vi "Main.vi"(11 "Module Admin":refnum<class "Delacor_lib_QMH_Module Admin.lvclass">) -> ()   [LabVIEW 2021, in "RT-AutoSequence.lvlib"]
doc: "This template is based off of the Queued Message Handler design pattern and the Queued Message Handler project template that ships with LabVIEW.\n\nThe main difference is that the queue is private to this module and communication between modules is performed via Broadcast and Request events.\n\nRequest events are wrapped in public API methods and are handled in the Event Handling Loop (EHL) of this VI. Any module can register for Broadcast events sent by this module. The EHL generates messages based on user interface actions.\n\nThe Message Handling Loop (MHL) processes messages generated by the EHL, or by other messages. The messages are string values, so new messages can be added easily to the Message Cases case structure in the MHL. Each message cluster can also provide an optional value for Message Data, which is a variant that can be converted to whatever message-specific data is required.\n_____\nBased on DQMH Project Template 7.0.1.1316."
uses:
  RT-AutoSequence.lvlib
  <vilib>/Delacor/Delacor QMH/Libraries/Module Admin_class/Delacor_lib_QMH_Module Admin.lvclass
  Module Data--cluster.ctl
  TCP Engine/Controls/TCP Engine I&O  Interupt Cluster.ctl
  <vilib>/Delacor/Delacor QMH/Libraries/Message Queue_class/Delacor_lib_QMH_Message Queue.lvclass/Delacor_lib_QMH_Message Queue.ctl
  Stop Argument--cluster.ctl
  <vilib>/Delacor/Delacor QMH/Libraries/Module Admin_class/Delacor_lib_QMH_Module Admin.lvclass/Delacor_lib_QMH_Module Admin.ctl
  Configuration Data Argument--cluster.ctl
  Start Auto Sequence Argument--cluster.ctl
  <vilib>/Utility/miscctls.llb/LVPointTypeDef.ctl
  <vilib>/Delacor/Delacor QMH/Libraries/Message Queue_class/Delacor_lib_QMH_Enqueue Message (Single).vi
  <vilib>/Delacor/Delacor QMH/Libraries/Module Admin_class/Delacor_lib_QMH_Get External Launch.vi
  <vilib>/Delacor/Delacor QMH/Libraries/Message Queue_class/Delacor_lib_QMH_Message Queue.lvclass
  TCP Engine/TCP Engine.lvlib
panel:
  out "Numeric":dbl
  out "error out":errorcluster
  out "Status":string
  in  "Simulate MHL Error":bool
  in  "Simulate EHL Error":bool
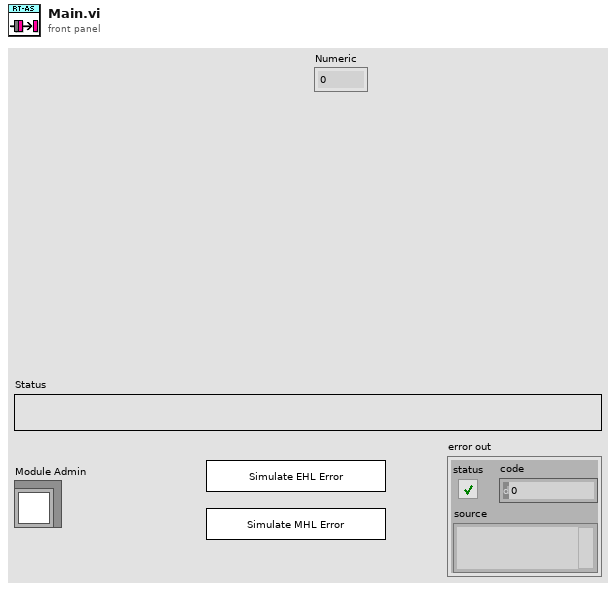
[diagram p1: front panel]
types:
  T1 = typedef "RT-AutoSequence.lvlib/Request Events--cluster.ctl" = cluster{"Stop Module":refnum<user-event>, "Show Panel":refnum<user-event>, "Hide Panel":refnum<user-event>, "Get Module Execution Status":refnum<user-event>, "Show Diagram":refnum<user-event>, "Configuration Data":refnum<user-event>, "Start Auto Sequence":refnum<user-event>}
  T2 = typedef "RT-AutoSequence.lvlib/Module Data--cluster.ctl" = cluster{"Status":string, "DO-Engine Interupt Q":refnum<queue>, "AS-Data's":cluster{"Physical Channel Name":string[], "Identification Name":string[], "Operation":bool[], "Time":dbl[]}, "Start Time":timestamp, "Config Received?":bool, "AS-Time Index":i32}
  T3 = enum32{"invalid lock state", "Not Locked", "Locked (No Password)", "Password-protected"}
  T4 = typedef "RT-AutoSequence.lvlib/Stop Argument--cluster.ctl" = cluster{"Origin":string, "Exit via Stop Module Req?":bool, "Wait for Module to stop?":bool}
  T5 = typedef "RT-AutoSequence.lvlib/Configuration Data Argument--cluster.ctl" = cluster{"AS-Configuration Data":variant}
  T6 = typedef "RT-AutoSequence.lvlib/Start Auto Sequence Argument--cluster.ctl" = cluster{"Start-AS":variant}
  T7 = typedef "LVPointTypeDef.ctl" = cluster{"Horizontal":i16, "Vertical":i16}
  T8 = enum32{"Invalid", "Standard", "Closed", "Hidden", "Minimized", "Maximized"}
  T9 = typedef "TCP Engine.lvlib/TCP Engine I&O  Interupt Cluster.ctl" = cluster{" Stop":bool, "JSON Variant":variant}
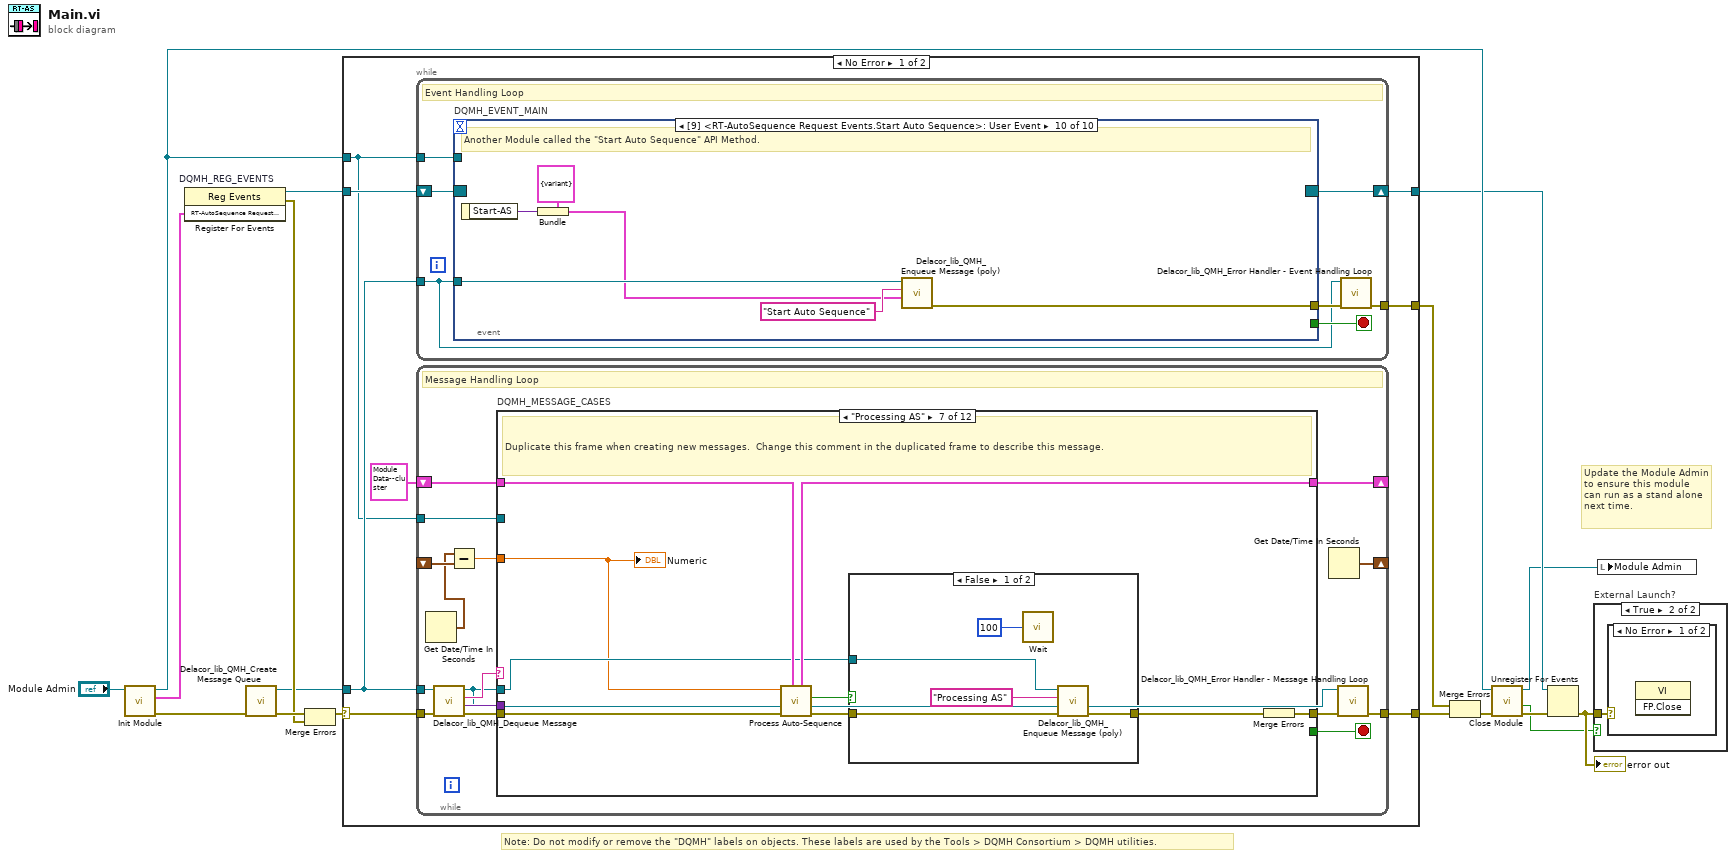
[diagram p0: block diagram]
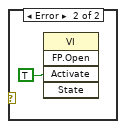
[diagram p3: hidden frame]
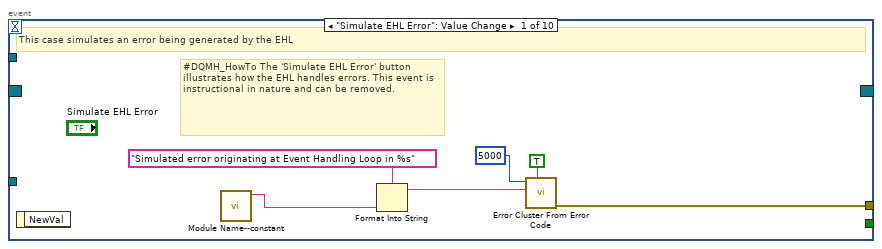
[diagram p4: hidden frame]
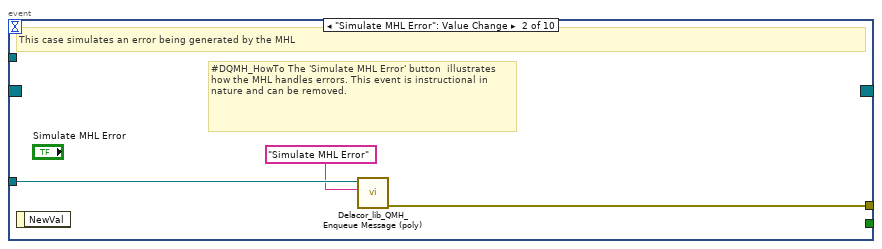
[diagram p5: hidden frame]
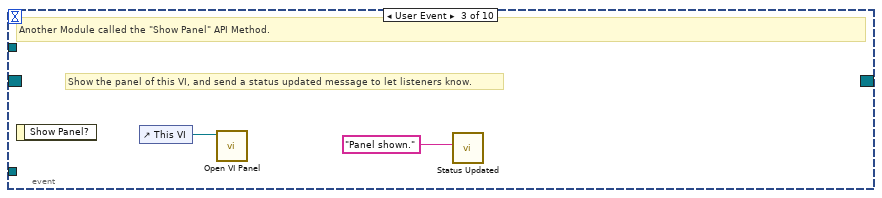
[diagram p6: hidden frame]
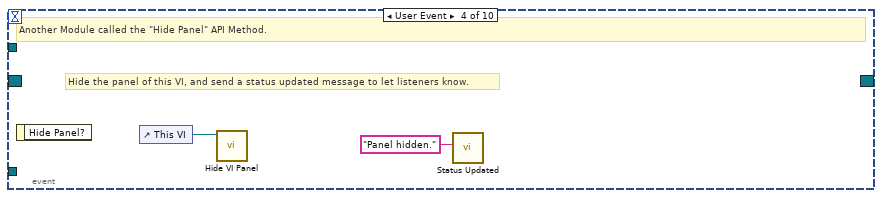
[diagram p7: hidden frame]
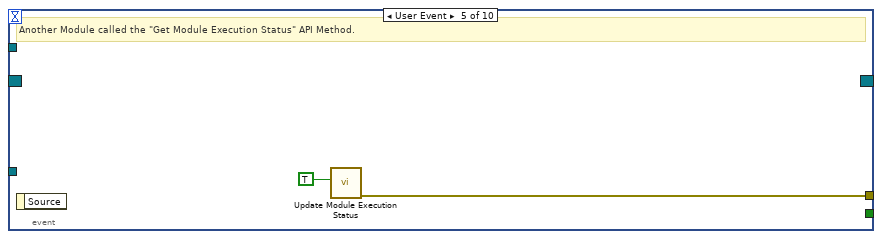
[diagram p8: hidden frame]
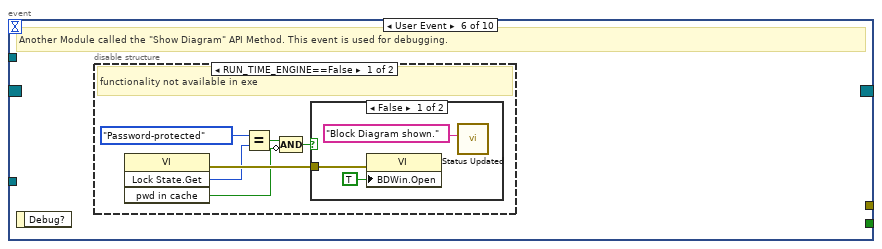
[diagram p9: hidden frame]
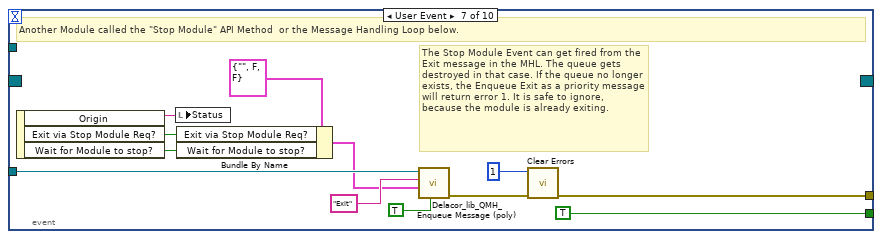
[diagram p12: hidden frame]
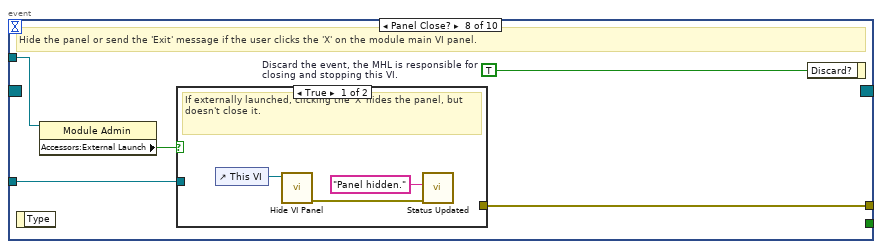
[diagram p13: hidden frame]
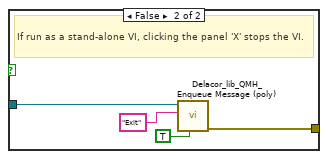
[diagram p14: hidden frame]
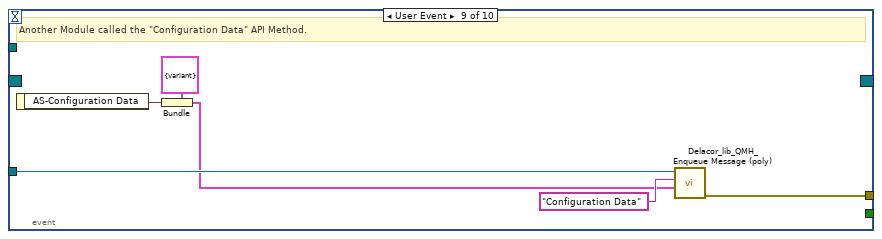
[diagram p15: hidden frame]
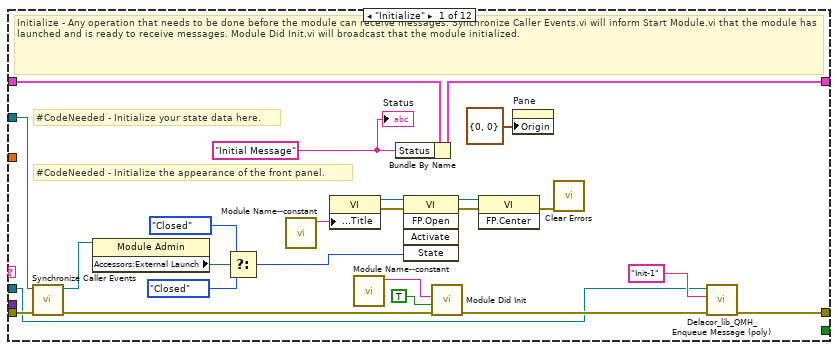
[diagram p16: hidden frame]
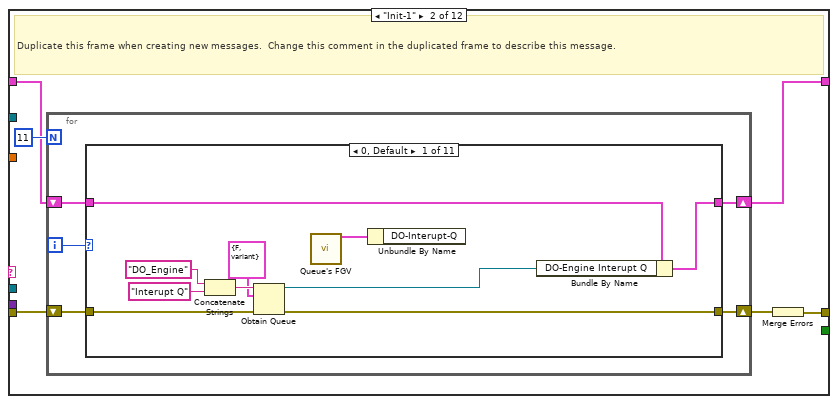
[diagram p17: hidden frame]
diagram:
  # "Note: Do not modify or remove the \"DQMH\" labels on objects. These labels are used by the Tools > DQMH Consortium > DQMH utilities."
  # "Update the Module Admin to ensure this module can run as a stand alone next time."
  n1 = call "Init Module.vi"("Singleton Module Admin in"="Module Admin") -> ("error out"=w16:errorcluster, "RT-AutoSequence Request Events"=w5:T1, "Singleton Module Admin out"=w8:refnum<class "Delacor_lib_QMH_Module Admin.lvclass">)  [unwired: 8 in]
  n2 = register-events "DQMH_REG_EVENTS"(w5) -> (reference out=w6:refnum<event-registration>, error out=w9:errorcluster)  [unwired: 2 in]
  n3 = call <vilib>:"Delacor_lib_QMH_Create Message Queue.vi"("error in"=w16) -> ("error out"=w11:errorcluster, "Message Queue"=w4:refnum<class "Delacor_lib_QMH_Message Queue.lvclass">)  [unwired: 9 in]
  n4 = Merge Errors(w11, w9) -> (w10:errorcluster)
  n5 = case shown="No Error" w10 {
    selector: w10 -> [w23 w276]
    tunnel: [w25 w275] -> w17
    tunnel: [w22 w274] -> w7
    tunnel: w6 -> [w21 w274]
    tunnel: w4 -> [w20 w269]
    tunnel: [w24 _] -> w14
    tunnel: w8 -> [w19 w270]
    frame No Error {
      n6 = while {
        tunnel: w20 -> [w26]
        shift-right: [w29] -> w22
        shift-left: w21 -> [w30]
        tunnel: [w31] -> w24
        tunnel: w19 -> [w27]
        stop <- w28 stop-if-true
        # "Event Handling Loop"
        n7 = event "DQMH_EVENT_MAIN" shown="[9] <RT-AutoSequence Request Events.Start Auto Sequence>: User Event" {
          selector: w30 -> [_ _ _ _ _ _ _ _ _ _]
          dyn-events: [_ _ _ _ _ _ _ _ _ _] -> w29
          timeout: _ -> [_ _ _ _ _ _ _ _ _ _]
          tunnel: [_ _ _ _ _ _ TRUE ("Discard?") _ _ _] -> w28
          tunnel: w26 -> [_ w40 _ _ _ _ w64 w71 w86 w92]
          tunnel: [w38 w41 _ _ w47 _ w67 w73 w81 w87] -> w32
          tunnel: w27 -> [_ _ _ _ _ _ _ w70 _ _]
          event "Simulate EHL Error": Value Change {
            # "#DQMH_HowTo The 'Simulate EHL Error' button  illustrates how the EHL handles errors. This event is instructional in nature and can be removed."
            # "This case simulates an error being generated by the EHL"
            n8 = event-data() -> ()  [unwired: 1 in, 1 out]
            n9 = call "Module Name--constant.vi"() -> ("Module Name"=w35:string)  [unwired: 11 in]
            n10 = Format Into String(format string="Simulated error originating at Event Handling Loop in %s", w35) -> (resulting string=w36:string)  [unwired: 2 in, 1 out]
            n11 = call <vilib>:"Error Cluster From Error Code.vi"("show call chain? (False)"=TRUE, "error message (\"\")"=w36, "error code (0)"=5000) -> ("error out"=w38:errorcluster)  [unwired: 6 in]
          }
          event "Simulate MHL Error": Value Change {
            # "#DQMH_HowTo The 'Simulate MHL Error' button  illustrates how the MHL handles errors. This event is instructional in nature and can be removed."
            # "This case simulates an error being generated by the MHL"
            n12 = event-data() -> ()  [unwired: 1 in, 1 out]
            n13 = call-poly <vilib>:"Delacor_lib_QMH_Enqueue Message (poly).vi"("Message"="Simulate MHL Error", "Message Queue in"=w40) -> ("error out"=w41:errorcluster)  [unwired: 8 in, 1 out]
          }
          event User Event {
            # "Show the panel of this VI, and send a status updated message to let listeners know."
            # "Another Module called the \"Show Panel\" API Method."
            n14 = event-data() -> ()  [unwired: 1 in, 1 out]
            n15 = control-ref of="This VI"() -> (w43:refnum<vi>)
            n16 = call "Open VI Panel.vi"("VI"=w43) -> ()  [unwired: 10 in, 1 out]
            n17 = call "Status Updated.vi"("Status"="Panel shown." ("format string")) -> ()  [unwired: 10 in, 1 out]
          }
          event User Event {
            # "Hide the panel of this VI, and send a status updated message to let listeners know."
            # "Another Module called the \"Hide Panel\" API Method."
            n18 = event-data() -> ()  [unwired: 1 in, 1 out]
            n19 = control-ref of="This VI"() -> (w45:refnum<vi>)
            n20 = call "Hide VI Panel.vi"("VI"=w45) -> ()  [unwired: 10 in, 1 out]
            n21 = call "Status Updated.vi"("Status"="Panel hidden." ("format string")) -> ()  [unwired: 10 in, 1 out]
          }
          event User Event {
            # "Another Module called the \"Get Module Execution Status\" API Method."
            n22 = event-data() -> ()  [unwired: 1 in, 1 out]
            n23 = call "Update Module Execution Status.vi"("Running?"=TRUE) -> ("error out"=w47:errorcluster)  [unwired: 10 in]
          }
          event User Event {
            # "Another Module called the \"Show Diagram\" API Method. This event is used for debugging."
            n24 = event-data() -> ()  [unwired: 1 in, 1 out]
            n25 = disable-structure shown="RUN_TIME_ENGINE==False" {
              frame condition #0 (active) {
                # "functionality not available in exe"
                n26 = invoke on="Invoke Node" class="VI" method="Lock State.Get"() -> (error out=w53:errorcluster, "Get Lock State"=w52:T3, "pwd in cache"=w49:bool)  [unwired: 4 in, 1 out]
                n27 = Equal?(x=T3."Password-protected", y=w52) -> (x = y?=w50:bool)
                n28 = Compound Arithmetic op=AND(w50, invert w49) -> (w48:bool)
                n29 = case shown="False" w48 {
                  tunnel: w53 -> [w56 _]
                  frame False {
                    n30 = property on="Property Node" class="VI"(error in=w56, "BDWin.Open"=TRUE ("Block Diagram Window:Open")) -> ()  [unwired: 1 in, 2 out]
                    n31 = call "Status Updated.vi"("Status"="Block Diagram shown." ("format string")) -> ()  [unwired: 10 in, 1 out]
                  }
                  frame True {
                    # "Password-protected VI, and the password is not in the cache. Do not show the diagram."
                  }
                }
              }
              frame condition #1 {
              }
            }
          }
          event User Event {
            # "The Stop Module Event can get fired from the Exit message in the MHL. The queue gets destroyed in that case. If the queue no longer exists, the Enqueue Exit as a priority message will return error 1. It is safe to ignore, because the module is already exiting."
            # "Another Module called the \"Stop Module\" API Method  or the Message Handling Loop below."
            n32 = event-data() -> ("Origin"=w63:string, "Exit via Stop Module Req?"=w59:bool, "Wait for Module to stop?"=w58:bool)  [unwired: 1 in]
            n33 = local write "Status"(w63) -> ()
            n34 = Bundle By Name(cluster=T4 {"Origin"="", "Exit via Stop Module Req?"=FALSE, "Wait for Module to stop?"=FALSE} ("Stop Argument"), "Exit via Stop Module Req?"=w59, "Wait for Module to stop?"=w58) -> (w57:T4)
            n35 = call-poly <vilib>:"Delacor_lib_QMH_Enqueue Message (poly).vi"("Priority Message? (F)"=TRUE, "Message Data"=w57, "Message"="Exit", "Message Queue in"=w64) -> ("error out"=w68:errorcluster)  [unwired: 6 in, 1 out]
            n36 = call <vilib>:"Clear Errors.vi"("error in (no error)"=w68, "specific error code to clear (0: all)"=1) -> ("error out"=w67:errorcluster)  [unwired: 4 in, 1 out]
          }
          event Panel Close? {
            w72 = TRUE  # Discard the event, the MHL is responsible for closing and stopping this VI.
            # "Hide the panel or send the 'Exit' message if the user clicks the 'X' on the module main VI panel."
            n37 = event-data() -> ()  [unwired: 1 in, 1 out]
            n38 = property on="Property Node" class="Module Admin"(reference=w70) -> ("Accessors:External Launch"=w69:bool)  [unwired: 1 in, 2 out]
            n39 = case shown="True" w69 {
              tunnel: w71 -> [_ w79]
              tunnel: [_ w80] -> w73
              frame True {
                # "If externally launched, clicking the 'X' hides the panel, but doesn't close it."
                n40 = control-ref of="This VI"() -> (w76:refnum<vi>)
                n41 = call "Hide VI Panel.vi"("VI"=w76) -> ("error out"=w74:errorcluster)  [unwired: 10 in]
                n42 = call "Status Updated.vi"("error in"=w74, "Status"="Panel hidden." ("format string")) -> ()  [unwired: 9 in, 1 out]
              }
              frame False {
                # "If run as a stand-alone VI, clicking the panel 'X' stops the VI."
                n43 = call-poly <vilib>:"Delacor_lib_QMH_Enqueue Message (poly).vi"("Priority Message? (F)"=TRUE, "Message"="Exit", "Message Queue in"=w79) -> ("error out"=w80:errorcluster)  [unwired: 7 in, 1 out]
              }
            }
            n44 = event-data ("Event Filter Node")("Discard?"=w72) -> ()  [unwired: 1 in, 1 out]
          }
          event User Event {
            # "Another Module called the \"Configuration Data\" API Method."
            n45 = event-data() -> ("AS-Configuration Data"=w82:variant)  [unwired: 1 in]
            n46 = Bundle(cluster=T5 {"AS-Configuration Data"=variant} ("Configuration Data Argument"), "AS-Configuration Data"=w82) -> (w83:T5)
            n47 = call-poly <vilib>:"Delacor_lib_QMH_Enqueue Message (poly).vi"("Message Data"=w83, "Message"="Configuration Data", "Message Queue in"=w86) -> ("error out"=w81:errorcluster)  [unwired: 7 in, 1 out]
          }
          event User Event {
            # "Another Module called the \"Start Auto Sequence\" API Method."
            n48 = event-data() -> ("Start-AS"=w88:variant)  [unwired: 1 in]
            n49 = Bundle(cluster=T6 {"Start-AS"=variant} ("Start Auto Sequence Argument"), "Start-AS"=w88) -> (w89:T6)
            n50 = call-poly <vilib>:"Delacor_lib_QMH_Enqueue Message (poly).vi"("Message Data"=w89, "Message"="Start Auto Sequence", "Message Queue in"=w92) -> ("error out"=w87:errorcluster)  [unwired: 7 in, 1 out]
          }
        }
        n51 = call-dynamic "Delacor_lib_QMH_Error Handler - Event Handling Loop.vi"("error in"=w32, "Message Queue in"=w26) -> ("dup error in"=w31:errorcluster)  [unwired: 8 in, 1 out]
      }
      n52 = while {
        tunnel: w20 -> [w97]
        shift-right: [w105] -> _
        shift-left: T2 {"Status"="", "DO-Engine Interupt Q"=refnum, "AS-Data's"={"Physical Channel Name"=[], "Identification Name"=[], "Operation"=[], "Time"=[]}, "Start Time"=timestamp(0 s since 1904-01-01), "Config Received?"=FALSE, "AS-Time Index"=0} ("Data Cluster") -> [w106]
        tunnel: w23 -> [w108]
        tunnel: [w100] -> w25
        tunnel: w19 -> [w101]
        shift-right: [w94] -> _
        shift-left: _ -> [w96]
        stop <- w104 stop-if-true
        # "Message Handling Loop"
        n53 = Get Date/Time In Seconds() -> (seconds since 1Jan1904=w93:timestamp)
        n54 = call-dynamic "Delacor_lib_QMH_Dequeue Message.vi"("error in"=w108, "Message Queue in"=w97) -> ("error out"=w107:errorcluster, "Message Data"=w102:variant, "Message"=w103:string, "Message Queue out"=w98:refnum<class "Delacor_lib_QMH_Message Queue.lvclass">)  [unwired: 6 in]
        n55 = Subtract(x=w93, y=w96) -> (x-y=w95:dbl)
        n56 = case "DQMH_MESSAGE_CASES" shown="\"Processing AS\"" w103 {
          selector: w103 -> [_ _ _ _ _ _ _ _ _ _ _ w264]
          tunnel: w98 -> [w109 _ _ _ w189 _ w203 _ _ w230 w252 _]
          tunnel: w107 -> [w130 w134 w175 w186 w197 w200 w207 w217 w226 w237 w258 w267]
          tunnel: [w110 w138 w175 w179 w187 w199 w209 w217 w225 w233 w253 w268] -> w99
          tunnel: w106 -> [w120 w136 w174 w178 w193 w198 w208 w216 w223 w232 w251 w265]
          tunnel: [w119 w133 w174 w182 w192 w198 w206 w216 w223 w232 w251 w265] -> w105
          tunnel: [_ _ _ _ _ _ _ _ _ _ w250 _] -> w104
          tunnel: w102 -> [_ _ _ w185 w196 _ _ _ _ w231 w249 _]
          tunnel: w101 -> [w121 _ _ _ _ _ _ _ _ w229 w244 _]
          tunnel: w95 -> [_ _ _ _ _ _ w201 _ _ _ _ _]
          frame "Initialize" {
            w115 = "Initial Message" ("Initial Message")
            # "#CodeNeeded - Initialize the appearance of the front panel."
            # "#CodeNeeded - Initialize your state data here."
            # "Initialize - Any operation that needs to be done before the module can receive messages. Synchronize Caller Events.vi will inform Start Module.vi that the module has launched and is ready to receive messages. Module Did Init.vi will broadcast that the module initialized."
            n57 = call "Synchronize Caller Events.vi"("error in"=w130, "Singleton Module Admin in"=w121) -> ("error out"=w129:errorcluster, "Singleton Module Admin out"=w116:refnum<class "Delacor_lib_QMH_Module Admin.lvclass">)  [unwired: 8 in]
            n58 = property on="Property Node" class="Module Admin"(reference=w116) -> ("Accessors:External Launch"=w125:bool)  [unwired: 1 in, 2 out]
            n59 = Select(t=T8."Closed" ("State"), s=w125, f=T8."Closed" ("State")) -> (s? t:f=w122:T8)
            n60 = call "Module Name--constant.vi"() -> ("Module Name"=w128:string)  [unwired: 11 in]
            n61 = property on="Property Node" class="VI"("Front Panel.Title"=w128) -> (reference out=w127:refnum<vi>, error out=w132:errorcluster)  [unwired: 2 in]
            n62 = call "Module Name--constant.vi"() -> ("Module Name"=w117:string)  [unwired: 11 in]
            n63 = Bundle By Name(cluster=w120, "Status"=w115) -> (w119:T2)
            n64 = invoke on="Invoke Node" class="VI" method="FP.Open"(reference=w127, error in=w132, "State"=w122) -> (reference out=w126:refnum<vi>, error out=w131:errorcluster)  [unwired: 2 in, 3 out]
            n65 = call "Module Did Init.vi"("error in"=w129, "Initialized?"=TRUE, "Origin"=w117) -> ("error out"=w111:errorcluster)  [unwired: 8 in]
            n66 = invoke on="Invoke Node" class="VI" method="FP.Center"(reference=w126, error in=w131) -> (error out=w113:errorcluster)  [unwired: 1 in, 2 out]
            n67 = property on="Pane" class="Pane"("Origin"=T7 {"Horizontal"=0, "Vertical"=0}) -> ()  [unwired: 2 in, 2 out]
            n68 = call <vilib>:"Clear Errors.vi"("error in (no error)"=w113) -> ()  [unwired: 5 in, 2 out]
            n69 = call-poly <vilib>:"Delacor_lib_QMH_Enqueue Message (poly).vi"("error in"=w111, "Message"="Init-1", "Message Queue in"=w109) -> ("error out"=w110:errorcluster)  [unwired: 7 in, 1 out]
            "Status" <- w115
          }
          frame "Init-1" {
            # "Duplicate this frame when creating new messages.  Change this comment in the duplicated frame to describe this message."
            n70 = for {
              N: 11 -> [_]
              shift-right: [w142] -> w133
              shift-left: w136 -> [w143]
              shift-right: [w140] -> w135
              shift-left: w134 -> [w139]
              i -> [w141]
              n71 = case shown="0, Default" w141 {
                tunnel: w143 -> [w147 w155 w157 w159 w161 w163 w165 w167 w169 w171 w173]
                tunnel: [w146 w155 w157 w159 w161 w163 w165 w167 w169 w171 w173] -> w142
                tunnel: [w148 w154 w156 w158 w160 w162 w164 w166 w168 w170 w172] -> w140
                tunnel: w139 -> [w149 w154 w156 w158 w160 w162 w164 w166 w168 w170 w172]
                frame 0, Default {
                  n72 = Concatenate Strings("DO_Engine" ("Engine Name"), "Interupt Q" ("string")) -> (w153:string)
                  n73 = Obtain Queue(name (unnamed)=w153, element data type=T9 {" Stop"=FALSE, "JSON Variant"=variant(string "")} ("I/O  Interupt Cluster"), error in (no error)=w149) -> (queue out=w144:refnum<queue>, error out=w148:errorcluster)  [unwired: 2 in, 1 out]
                  n74 = call "Queue's FGV.vi"() -> ("Cluster"=w145:cluster{"DO-Interupt-Q":refnum<queue>})  [unwired: 14 in, 1 out]
                  n75 = Unbundle By Name(w145) -> ()  [unwired: 1 out]
                  n76 = Bundle By Name(cluster=w147, "DO-Engine Interupt Q"=w144) -> (w146:T2)
                }
                frame 1 {
                }
                frame 2 {
                }
                frame 3 {
                }
                frame 4 {
                }
                frame 5 {
                }
                frame 6 {
                }
                frame 7 {
                }
                frame 8 {
                }
                frame 9 {
                }
                frame 10 {
                }
              }
            }
            n77 = Merge Errors(w135) -> (w138:errorcluster)
          }
          frame "---Module Specific---" {
            # "Separator -- The following cases handle messages specific to this Module."
          }
          frame "Configuration Data" {
            # "This Request event will send the AutoSequence configuration which has been received from the Host through TCP-IP module to AutoSequence Module."
            n78 = Variant To Data(error in=w186, type=T5 {"AS-Configuration Data"=variant} ("Configuration Data Argument"), Variant=w185) -> (data=w183:T5, error out=w180:errorcluster)
            n79 = Unbundle By Name(w183) -> ("AS-Configuration Data"=w181:variant)
            n80 = Bundle By Name(cluster=w178, "Config Received?"=TRUE) -> (w177:T2)
            n81 = call "Configure Timing's.vi"("Data Cluster In"=w177, "error in (no error)"=w180, "Configuration Data"=w181) -> ("error out"=w179:errorcluster, "Data Cluster Out"=w182:T2)  [unwired: 7 in]
          }
          frame "Start Auto Sequence" {
            # "This Request Event will give the start command which has been received from the Host using TCP-IP module to the Auto Sequence Module."
            n82 = Variant To Data(error in=w197, type=T6 {"Start-AS"=variant} ("Start Auto Sequence Argument"), Variant=w196) -> (data=w194:T6, error out=w188:errorcluster)
            n83 = Unbundle By Name(w194) -> ()  [unwired: 1 out]
            n84 = call-poly <vilib>:"Delacor_lib_QMH_Enqueue Message (poly).vi"("error in"=w188, "Message"="Processing AS", "Message Queue in"=w189) -> ("error out"=w187:errorcluster)  [unwired: 7 in, 1 out]
            n85 = Get Date/Time In Seconds() -> (seconds since 1Jan1904=w191:timestamp)
            n86 = Bundle By Name(cluster=w193, "Start Time"=w191) -> (w192:T2)
          }
          frame "---Copy This Frame---" {
            # "Duplicate this frame when creating new messages.  Change this comment in the duplicated frame to describe this message."
            n87 = Merge Errors(w200) -> (w199:errorcluster)
          }
          frame "Processing AS" {
            # "Duplicate this frame when creating new messages.  Change this comment in the duplicated frame to describe this message."
            n88 = call "Process Auto-Sequence.vi"("Data Cluster In"=w208, "error in"=w207, "y"=w201) -> ("error out"=w204:errorcluster, "Again Process?"=w205:bool, "Data Cluster Out"=w206:T2)  [unwired: 6 in]
            n89 = case shown="False" w205 {
              tunnel: w204 -> [w213 w215]
              tunnel: w203 -> [w214 _]
              tunnel: [w212 w215] -> w202
              frame False {
                n90 = call "Wait"("Count(mSec)"=u32 100 ("milliseconds to wait")) -> ()  [unwired: 1 out]
                n91 = call-poly <vilib>:"Delacor_lib_QMH_Enqueue Message (poly).vi"("error in"=w213, "Message"="Processing AS", "Message Queue in"=w214) -> ("error out"=w212:errorcluster)  [unwired: 7 in, 1 out]
              }
              frame True {
              }
            }
            n92 = Merge Errors(w202) -> (w209:errorcluster)
            "Numeric" <- w201
          }
          frame "---Exit and Error Handling---" {
            # "Separator - The following cases handle errors and exit messages."
          }
          frame "Simulate MHL Error" {
            # "#DQMH_HowTo The 'Simulate MHL Error' button  illustrates how the MHL handles errors. This event is instructional in nature and can be removed."
            # "Simulate an error occurring at the MHL"
            n93 = call "Module Name--constant.vi"() -> ("Module Name"=w219:string)  [unwired: 11 in]
            n94 = Format Into String(format string="Simulated error originating at Message Handling Loop in %s", w219) -> (resulting string=w220:string)  [unwired: 2 in, 1 out]
            n95 = call <vilib>:"Error Cluster From Error Code.vi"("show call chain? (False)"=TRUE, "error message (\"\")"=w220, "error code (0)"=5001) -> ("error out"=w224:errorcluster)  [unwired: 6 in]
            n96 = Merge Errors(w226, w224) -> (w225:errorcluster)
          }
          frame "Error" {
            # "#CodeRecommended - If the module is running in standalone mode (External Launch = FALSE), this code will pop up an error dialog and call the 'Exit' message if an error occurs. Add more fine-grained error management here."
            # "Error - Check the error message data and respond accordingly. This message is sent by the \"Error Handler\" VIs at the end of each loop in this application."
            n97 = property on="Property Node" class="Module Admin"(reference=w229) -> ("Accessors:External Launch"=w228:bool)  [unwired: 1 in, 2 out]
            n98 = Variant To Data(error in=w237, type=errorcluster {"status"=FALSE, "code"=0, "source"=""} ("error constant"), Variant=w231) -> (data=w227:errorcluster, error out=w235:errorcluster)
            n99 = local write "error out"(w227) -> ()
            n100 = call "Error Reported.vi"("Error"=w227) -> ()  [unwired: 10 in, 1 out]
            n101 = case shown="False" w228 {
              tunnel: [w242 _] -> w234
              tunnel: w230 -> [w240 _]
              tunnel: w227 -> [w241 _]
              frame False {
                n102 = disable-structure shown="Default" {
                  disable-tunnel: w241 -> [w243 _]
                  frame condition #0 (active) {
                    # "If the module is running standalone, then pop up an error dialog and call the \"Exit\" message."
                    n103 = call <vilib>:"Simple Error Handler.vi"("error in (no error)"=w243) -> ()  [unwired: 4 in, 5 out]
                  }
                  frame condition #1 {
                    # "To prevent the Simple Error Handler VI from being loaded (e.g. when deploying to a Real-Time target), add the Conditional Disable Symbol \"DQMH_Disable_SEH\" to your project and set it to TRUE."
                  }
                }
                n104 = call-poly <vilib>:"Delacor_lib_QMH_Enqueue Message (poly).vi"("Priority Message? (F)"=TRUE, "Message"="Exit", "Message Queue in"=w240) -> ("error out"=w242:errorcluster)  [unwired: 7 in, 1 out]
              }
              frame True {
                # "If the module was launched externally, calling the Error Reported broadcast VI is the only action performed by the \"Error\" message. The module's caller can then process the error appropriately."
              }
            }
            n105 = Merge Errors(w235, w234) -> (w233:errorcluster)
          }
          frame "Exit" {
            w248 = 91  # 91: not all Exit messages will have an argument
            w250 = TRUE  # Stop the VI
            # "Release the message queue reference"
            # "#CodeNeeded - Add any required cleanup code here."
            # "Exit - Exit the application."
            n106 = Variant To Data(error in=w258, type=T4 {"Origin"="", "Exit via Stop Module Req?"=FALSE, "Wait for Module to stop?"=FALSE} ("Stop Argument"), Variant=w249) -> (data=w246:T4, error out=w255:errorcluster)
            n107 = call <vilib>:"Clear Errors.vi"("error in (no error)"=w255, "specific error code to clear (0: all)"=w248) -> ("error out"=w257:errorcluster)  [unwired: 4 in, 1 out]
            n108 = control-ref of="This VI"() -> (w245:refnum<vi>)
            n109 = call-dynamic "Delacor_lib_QMH_Release Message Queue.vi"("error in"=w257, "Message Queue"=w252) -> ("error out"=w256:errorcluster)  [unwired: 9 in]
            n110 = call "Handle Exit.vi"("Stop Argument"=w246, "Admin in"=w244, "VI reference"=w245) -> ("error out"=w254:errorcluster)  [unwired: 7 in, 1 out]
            n111 = Merge Errors(w256, w254) -> (w253:errorcluster)
            n112 = call "Error Reported.vi"("Error"=w253) -> ()  [unwired: 10 in, 1 out]
          }
          frame Default {
            # "'Default' case only runs if there is a message that isn't defined in any of the other cases.  Output a programming error."
            n113 = call "Module Name--constant.vi"() -> ("Module Name"=w263:string)  [unwired: 11 in]
            n114 = Format Into String(format string="The invalid message string \"%s\" was received in the Message Handling Loop for module \"%s\".", w264, w263) -> (resulting string=w259:string)  [unwired: 2 in, 1 out]
            n115 = call <vilib>:"Error Cluster From Error Code.vi"("show call chain? (False)"=TRUE, "error message (\"\")"=w259, "error code (0)"=1) -> ("error out"=w266:errorcluster)  [unwired: 6 in]
            n116 = Merge Errors(w267, w266) -> (w268:errorcluster)
          }
        }
        n117 = Get Date/Time In Seconds() -> (seconds since 1Jan1904=w94:timestamp)
        n118 = call-dynamic "Delacor_lib_QMH_Error Handler - Message Handling Loop.vi"("error in"=w99, "Message Queue in"=w98) -> ("dup error in"=w100:errorcluster)  [unwired: 8 in, 1 out]
      }
    }
    frame Error {
      # "Synchronize Caller Events.vi will inform Start Module.vi that the module has launched and will let the code calling Start Module.vi register for broadcasts and would permit the caller receive the broadcast that an error occurred at launch time."
      n119 = call-dynamic "Delacor_lib_QMH_Release Message Queue.vi"("error in"=w276, "Message Queue"=w269) -> ("error out"=w275:errorcluster)  [unwired: 9 in]
      n120 = call "Synchronize Caller Events.vi"("Singleton Module Admin in"=w270) -> ("error out"=w277:errorcluster)  [unwired: 9 in, 1 out]
      n121 = call "Module Name--constant.vi"() -> ("Module Name"=w273:string)  [unwired: 11 in]
      n122 = Format Into String(format string="An error occurred during initialization. %s is no longer running.", w273) -> (resulting string=w271:string)  [unwired: 2 in, 1 out]
      n123 = Merge Errors(w275, w277) -> (w278:errorcluster)
      n124 = call "Error Reported.vi"("Additional Information"=w271, "Error"=w278) -> ()  [unwired: 9 in, 1 out]
    }
  }
  n125 = Merge Errors(w14, w17) -> (w13:errorcluster)
  n126 = call "Close Module.vi"("error in"=w13, "Module Admin in"=w8) -> ("error out"=w15:errorcluster, "External Launch"=w1:bool, "Module Admin out"=w2:refnum<class "Delacor_lib_QMH_Module Admin.lvclass">)  [unwired: 7 in]
  n127 = Unregister For Events(event registration refnum=w7, error in=w15) -> (error out=w12:errorcluster)
  "error out" <- w12
  n128 = case "External Launch?" shown="True" w1 {
    tunnel: w12 -> [_ w279]
    frame False {
    }
    frame True {
      n129 = case shown="No Error" w279 {
        frame No Error {
          n130 = invoke on="Invoke Node" class="VI" method="FP.Close"() -> ()  [unwired: 3 in, 3 out]
        }
        frame Error {
          n131 = invoke on="Invoke Node" class="VI" method="FP.Open"("Activate"=TRUE ("Activate?")) -> ()  [unwired: 4 in, 5 out]
        }
      }
    }
  }
  n132 = local write "Module Admin"(w2) -> ()
